vi "Double Gaussian fitting model.vi"(3 "output control":T1 caption="输出控制", 4 "data":variant caption="数据", 5 "X":dbl[](array[numeric]), 6 "a":dbl[](array[numeric])) -> (0 "error out":errorcluster caption="错误输出", 1 "f'(X,a)":dbl[][](array[numeric]), 2 "f(X,a)":dbl[](array[numeric]))   [LabVIEW 2013]
doc: "This template is the starting point for creating a model function to be passed to the Nonlinear Curve Fit.vi."
uses:
  <vilib>/gmath/NumericalOptimization/LM_output select.ctl
  <vilib>/gmath/NI_Gmath.lvlib
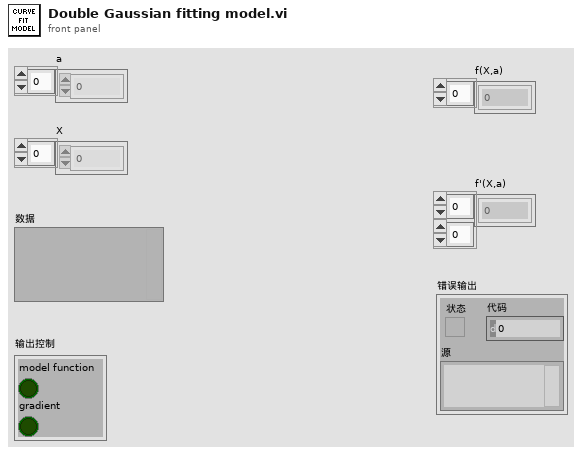
[diagram p1: front panel]
types:
  T1 = typedef "NI_Gmath.lvlib/LM_output select.ctl" = cluster{"model function":bool, "gradient":bool}
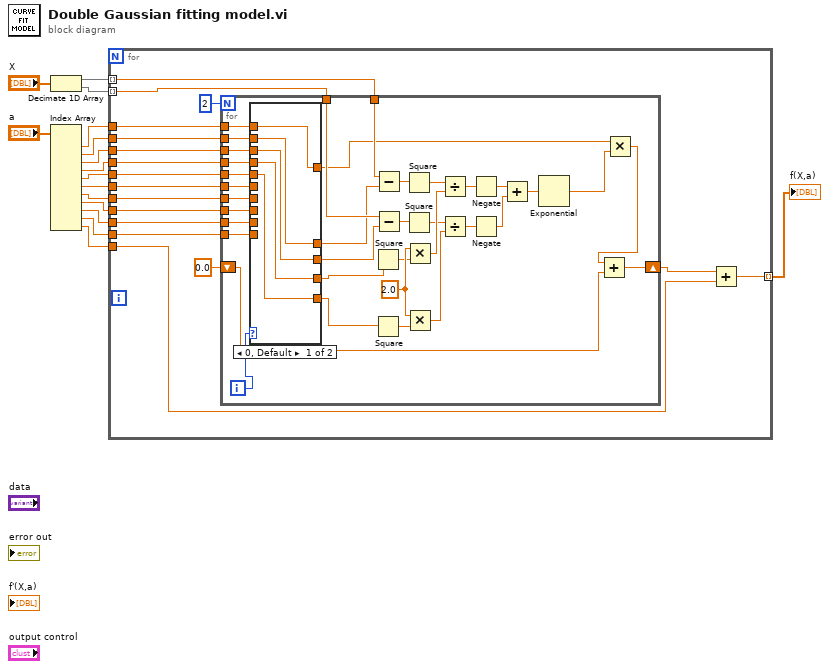
[diagram p0: block diagram]
diagram:
  n1 = Decimate 1D Array("X") -> (w8:dbl[], w7:dbl[])
  n2 = Index Array(array="a") -> (element #1=w15:dbl, element #2=w14:dbl, element #3=w13:dbl, element #4=w12:dbl, element #5=w11:dbl, element #6=w9:dbl, element #7=w6:dbl, element #8=w5:dbl, element #9=w4:dbl, element #10=w3:dbl, element #11=w2:dbl)  [unwired: 11 in]
  n3 = for {
    tunnel: w15 -> [w32]
    tunnel: w14 -> [w31]
    tunnel: w13 -> [w30]
    tunnel: w12 -> [w29]
    tunnel: w11 -> [w28]
    tunnel: w7 -> [w21] mode=indexing
    tunnel: w9 -> [w27]
    tunnel: w8 -> [w22] mode=indexing
    tunnel: w6 -> [w26]
    tunnel: w5 -> [w25]
    tunnel: w4 -> [w24]
    tunnel: w3 -> [w23]
    tunnel: w2 -> [w19]
    tunnel: [w17] -> w1 mode=indexing
    n4 = for {
      N: 2 -> [_]
      tunnel: w32 -> [w54]
      tunnel: w31 -> [w53]
      tunnel: w30 -> [w52]
      tunnel: w29 -> [w51]
      tunnel: w28 -> [w50]
      tunnel: w27 -> [w49]
      tunnel: w26 -> [w48]
      tunnel: w25 -> [w47]
      tunnel: w24 -> [w46]
      tunnel: w23 -> [w45]
      tunnel: w22 -> [w44]
      tunnel: w21 -> [w43]
      shift-right: [w35] -> w18
      shift-left: 0.0 -> [w34]
      i -> [w55]
      w67 = 2.0 ("x")
      n5 = case shown="0, Default" w55 {
        tunnel: w54 -> [w74 _]
        tunnel: w53 -> [w73 _]
        tunnel: w52 -> [w72 _]
        tunnel: w51 -> [w71 _]
        tunnel: w50 -> [w70 _]
        tunnel: w49 -> [_ w75]
        tunnel: w48 -> [_ w76]
        tunnel: w47 -> [_ w77]
        tunnel: w46 -> [_ w78]
        tunnel: w45 -> [_ w79]
        tunnel: [w73 w76] -> w42
        tunnel: [w72 w77] -> w41
        tunnel: [w71 w78] -> w40
        tunnel: [w70 w79] -> w39
        tunnel: [w74 w75] -> w37
        frame 0, Default {
        }
        frame 1 {
        }
      }
      n6 = Square(x=w40) -> (x^2=w66:dbl)
      n7 = Square(x=w39) -> (x^2=w65:dbl)
      n8 = Subtract(x=w44, y=w42) -> (x-y=w69:dbl)
      n9 = Subtract(x=w43, y=w41) -> (x-y=w68:dbl)
      n10 = Square(x=w69) -> (x^2=w64:dbl)
      n11 = Square(x=w68) -> (x^2=w62:dbl)
      n12 = Multiply(x=w67, y=w66) -> (x*y=w63:dbl)
      n13 = Multiply(x=w67, y=w65) -> (x*y=w61:dbl)
      n14 = Divide(x=w64, y=w63) -> (x/y=w60:dbl)
      n15 = Divide(x=w62, y=w61) -> (x/y=w59:dbl)
      n16 = Negate(x=w60) -> (-x=w58:dbl)
      n17 = Negate(x=w59) -> (-x=w57:dbl)
      n18 = Add(x=w58, y=w57) -> (x+y=w56:dbl)
      n19 = Exponential(1:w56) -> (0:w38:dbl)
      n20 = Multiply(x=w37, y=w38) -> (x*y=w36:dbl)
      n21 = Add(x=w36, y=w34) -> (x+y=w35:dbl)
    }
    n22 = Add(x=w18, y=w19) -> (x+y=w17:dbl)
  }
  "f(X,a)" <- w1
